vi "GateSTS v2.vi"(5 "Store\nSecond Gate?":bool=TRUE, 6 "Attributes":string[][](array[string]), 7 "Increment Gate (V)":dbl, 8 "End Gate (V)":dbl, 9 "Start Gate (V)":dbl, 10 "Basename":string) -> (3 "Stop Loop":bool)   [LabVIEW 2021]
uses:
  <userlib>/Nanonis Prog Interface V5/Nanonis Prog Interface.lvlib
panel:
  in  "Tabs":T1(tab)
  in  "Sweep second gate?":bool
  out "Sweep time (min)":dbl
  in  "Nanonis LI      Ext LI":bool=TRUE
  in  "Single spectrum?":bool
  in  "Time Constant (s)":T2(ring)=enum."10 ms"
  in  "Frequency (Hz)":dbl=1541.2 format="%#_6p"
  in  "End Bias (V)":dbl=0.04 format="%#_6p"
  in  "Start Bias (V)":dbl=-0.04 format="%#_6p"
  in  "Energy resolution (V)":dbl=0.001 format="%#_6p"
  in  "Stop":bool
  out "Current Gate Voltage (V)":dbl
  in  "?":bool
  out "HDF5 DATANAME":string
  in  "Run lockin?":bool=TRUE
  in  "Store\nLock-in\nParameters?":bool=TRUE
  in  "Store\nTemperatures?":bool
  in  "Store\nMagnetic Field?":bool
  in  "Zigzag Raster?":bool
  in  "Insert Loop Index\ninto Basename?":bool
  in  "Loop Forever?":bool
  out "Loop Index":i32
  in  "Loop Index Offset":i32=1
  in  "Make .dat files?":bool=TRUE
  out "Ender":bool
  # "Gate STS"
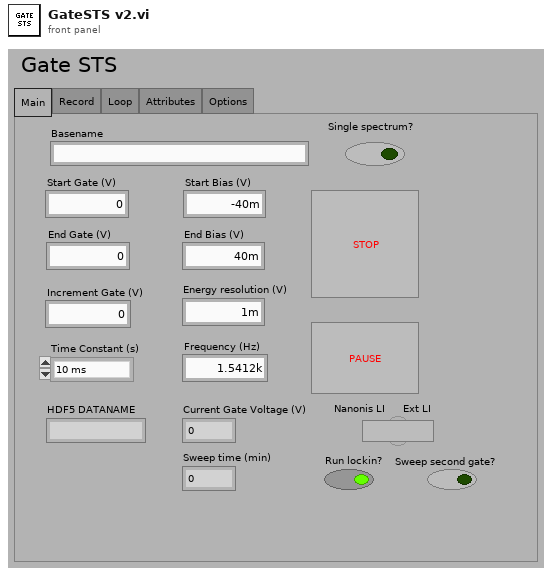
[diagram p1: front panel]
types:
  T1 = enum32{"Main", "Record", "Loop", "Attributes", "Options"}
  T2 = enum16{"10 us", "30 us", "100 us", "300 us", "1 ms", "3 ms", "10 ms", "30 ms", "100 ms", "300 ms", "1 s", "3 s", "10 s", "30 s", "100 s", "300 s", "1 ks", "3 ks", "10 ks", "30 ks"}
  T3 = enum16{"Set Amplitude", "Get Amplitude", "Set Frequency", "Get Frequency", "Set Harmonic", "Get Harmonic", "Set Phase", "Get Phase", "Auto Phase", "Add to Phase", "Autogain", "Set Time Constant", "Get Time Constant", "Set Sensitivity", "Get Sensitivity", "Set Input A", "Set Input A-B", "Get Input Setting", "Set Offset", "Get Offset"}
  T4 = cluster{"Save all":enum16{"no change", "on", "off"}, "Number of Sweeps (0=no change)":i32}
  T5 = enum16{"Set Voltage", "Read Voltage", "Read Current", "Output On", "Output Off", "Set Increment", "Set Increment Time", "Stop Voltage Set", "Set Maximum Voltage", "Get Maximum Voltage"}
  T6 = enum16{"Output 2 (V)", "Output 3 (V)", "Output 4 (V)"}
  T7 = enum16{"Read State", "Hold", "Ramp to Set", "Ramp to Zero", "Read Switch Heater", "Switch Heater On", "Switch Heater Off", "Read Voltage", "Read Current", "Read Field", "Read Persistent Field", "Read Target Field", "Set Target Field", "Read Ramp Rate", "Set Ramp Rate"}
  T8 = enum16{"pot_temp", "sorb_temp", "needle_valve_temp", "still_temp", "mix_chamber_temp", "stm_rx_temp", "stm_cx_temp", "tank_pressure", "condense_pressure", "still_pressure", "turbo_back_pressure", "n2_trap_pressure"}
  T9 = enum16{"Set Amplitude", "Get Amplitude", "Set Frequency", "Get Frequency", "Set Harmonic", "Get Harmonic", "Set Phase", "Get Phase", "Auto Phase", "Add to Phase", "Autogain", "Set Time Constant", "Get Time Constant", "Set Sensitivity", "Get Sensitivity", "Set Input A", "Set Input A-B", "Get Input Setting", "Set Offset", "Get Offset"}[]
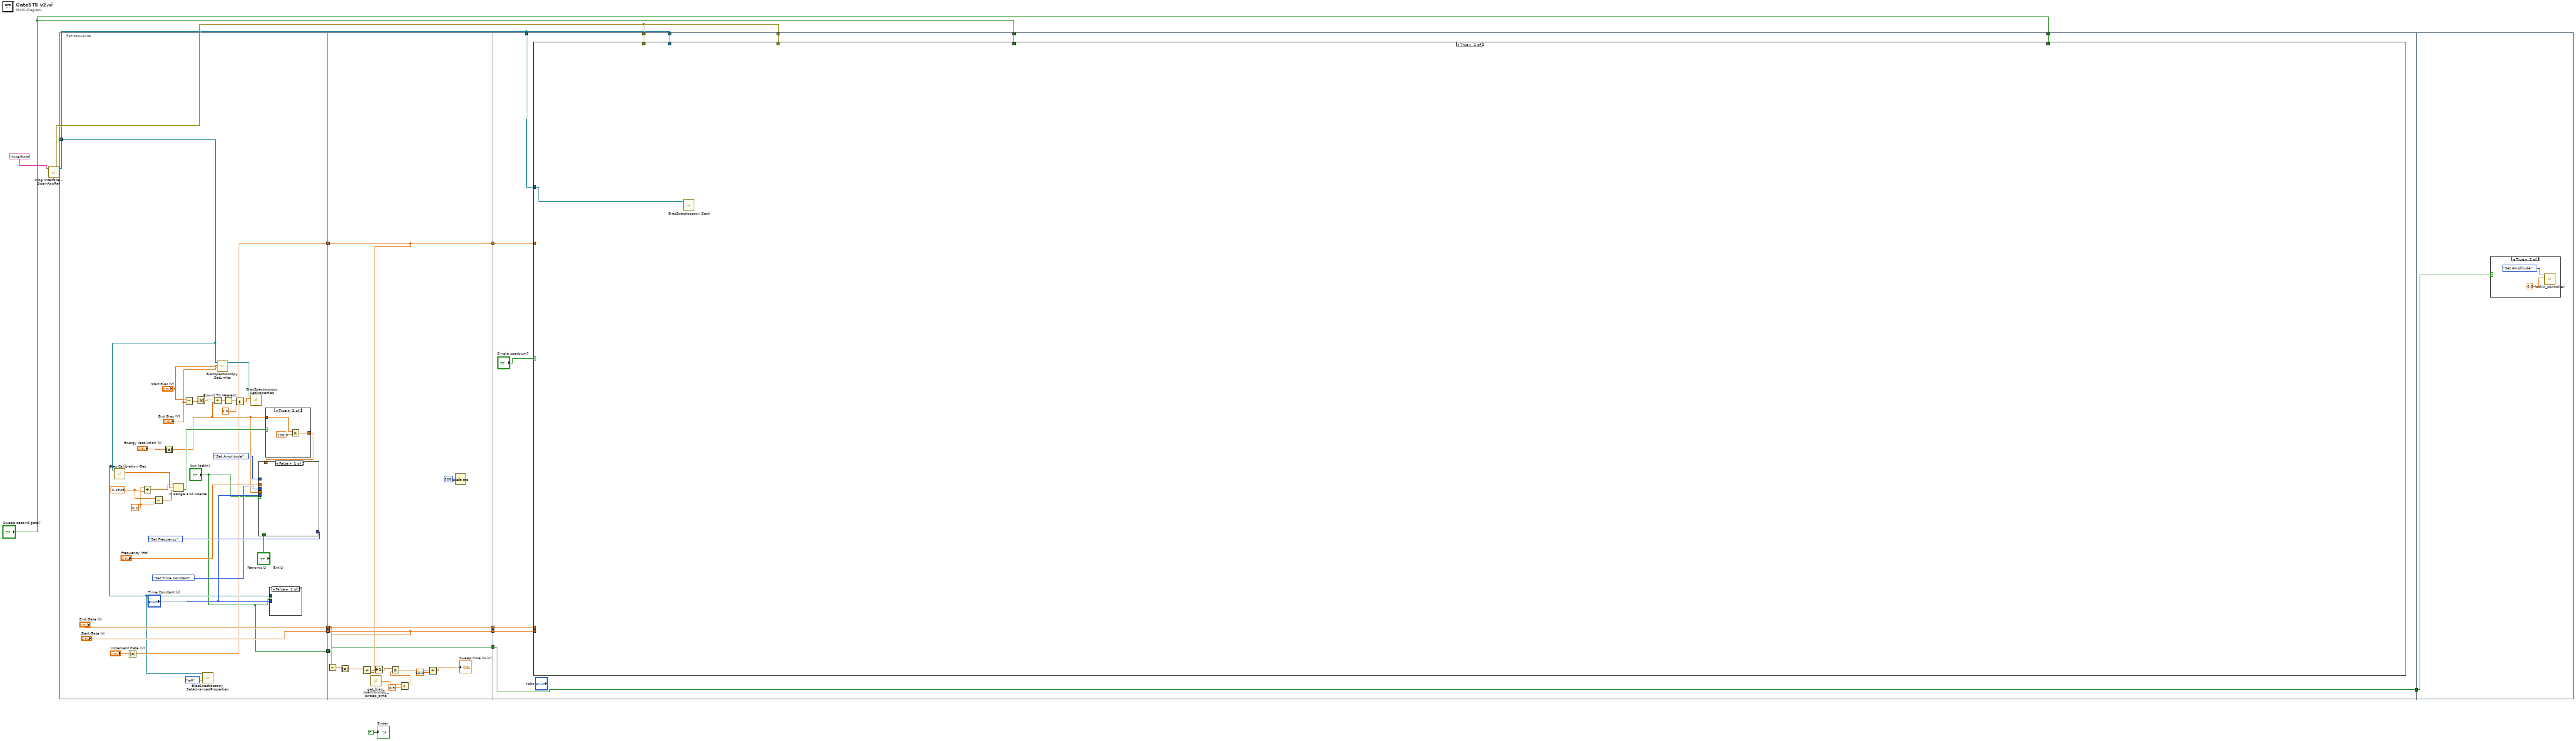
[diagram p0: block diagram]
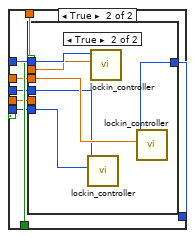
[diagram p2: hidden frame]
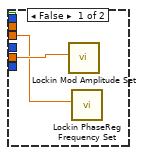
[diagram p3: hidden frame]
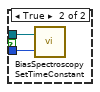
[diagram p4: hidden frame]
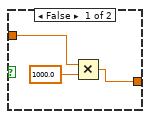
[diagram p5: hidden frame]
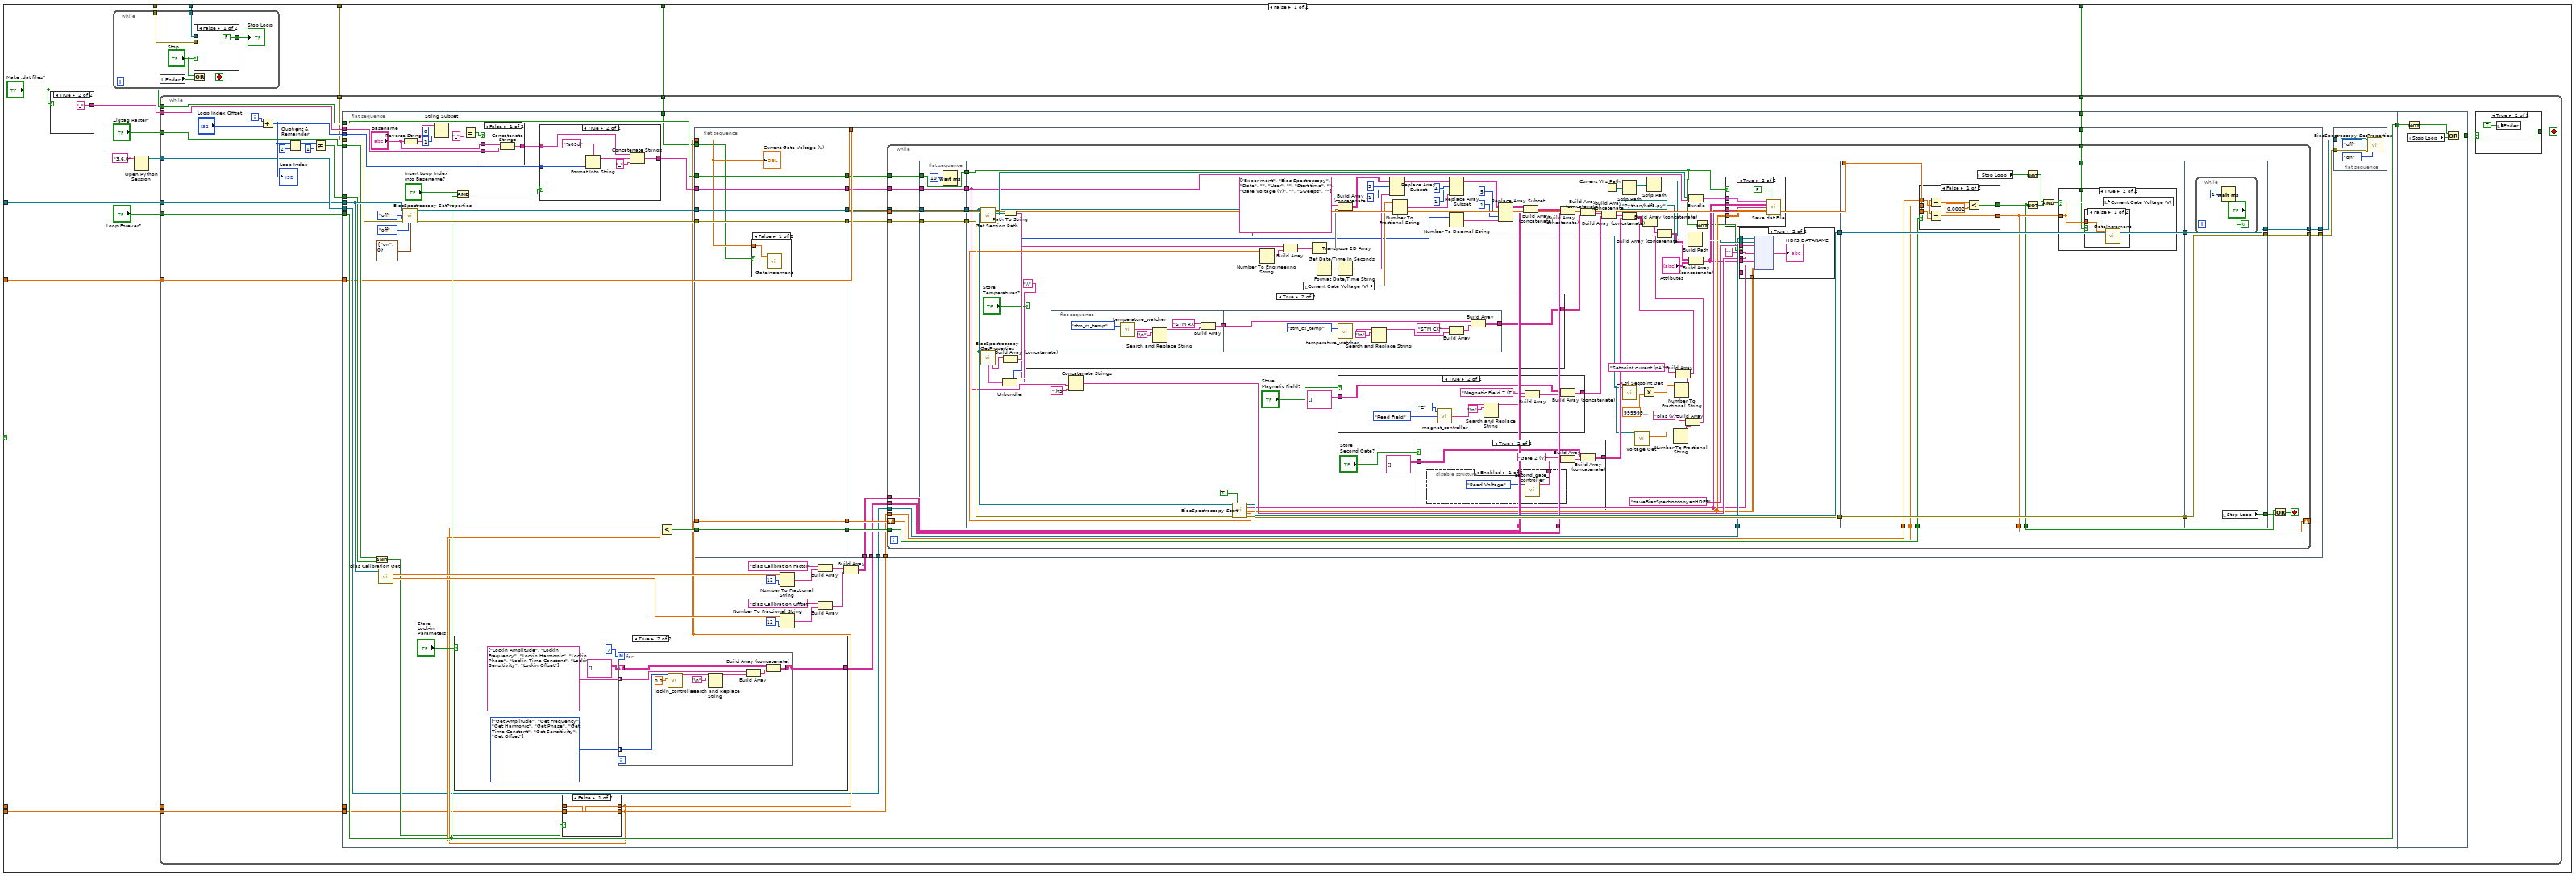
[diagram p6: hidden frame]
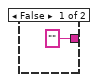
[diagram p7: hidden frame]
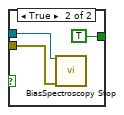
[diagram p8: hidden frame]
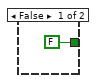
[diagram p9: hidden frame]
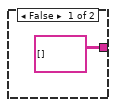
[diagram p13: hidden frame]
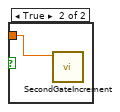
[diagram p14: hidden frame]
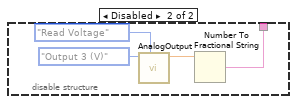
[diagram p17: hidden frame]
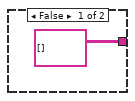
[diagram p20: hidden frame]
diagram:
  n1 = call <userlib>:"Prog Interface - OpenAppRef.vi"("Machine name (local machine IP)"="localhost" ("machine name (localhost)")) -> ("Error out"=w12:errorcluster, "Application reference"=w11:refnum<vi>)  [unwired: 5 in]
  n2 = flat-sequence {
    tunnel: w11 -> [w17]
    tunnel: ["End Gate (V)"] -> w9
    tunnel: ["Start Gate (V)"] -> w7
    tunnel: [w20] -> w5
    tunnel: ["Run lockin?"] -> w3
    tunnel: [w73] -> w10
    tunnel: w9 -> [w73]
    tunnel: [w72] -> w8
    tunnel: w7 -> [w72]
    tunnel: [w74] -> w6
    tunnel: w5 -> [w74]
    tunnel: w3 -> [w70]
    tunnel: [w70] -> w2
    tunnel: w12 -> [w95]
    tunnel: w12 -> [w94]
    tunnel: w11 -> [w93]
    tunnel: w11 -> [w92]
    tunnel: w10 -> [w90]
    tunnel: w8 -> [w89]
    tunnel: w6 -> [w88]
    tunnel: "Sweep second gate?" -> [w87]
    tunnel: "Sweep second gate?" -> [w86]
    tunnel: w2 -> [w85]
    tunnel: [w85] -> w1
    tunnel: w1 -> [w465]
    frame #0 {
      w38 = 0.1 ("y")
      w39 = 0.4945 ("x")
      n3 = call <userlib>:"Bias Calibration Get.vi"("Application ref in"=w17) -> ("Calibration (V/V)"=w41:sgl)  [unwired: 7 in, 3 out]
      n4 = Absolute Value(x="Increment Gate (V)") -> (abs(x)=w20:dbl)
      n5 = Add(x=w39, y=w38) -> (x+y=w40:dbl)
      n6 = Subtract(x=w39, y=w38) -> (x-y=w37:dbl)
      n7 = Absolute Value(x="Energy resolution (V)") -> (abs(x)=w22:dbl)
      n8 = In Range and Coerce(upper limit=w40, x=w41, lower limit=w37) -> (In Range?=w36:bool)  [unwired: 1 out]
      n9 = Subtract(x="Start Bias (V)", y="End Bias (V)") -> (x-y=w45:dbl)
      n10 = Absolute Value(x=w45) -> (abs(x)=w44:dbl)
      n11 = call <userlib>:"BiasSpectroscopy SetAdvancedProperties.vi"("Application ref in"=w17, "Lockin run (no change)"=enum16{"no change", "on", "off"}."off") -> ()  [unwired: 12 in, 2 out]
      n12 = Divide(x=w44, y=w22) -> (x/y=w43:dbl)
      n13 = call <userlib>:"BiasSpectroscopy SetLimits.vi"("End value (V)"="End Bias (V)", "Start value (V)"="Start Bias (V)", "Application ref in"=w17) -> ("Application ref out"=w42:refnum<vi>)  [unwired: 5 in, 1 out]
      n14 = Round To Nearest(number=w43) -> (nearest integer value=w33:dbl)
      n15 = Add(x=w33, y=1.0) -> (x+y=w31:dbl)
      n16 = call <userlib>:"BiasSpectroscopy SetProperties.vi"("Application ref in"=w42, "Number of points (0=no change)"=w31) -> ()  [unwired: 12 in, 2 out]
      n17 = case shown="True" w36 {
        tunnel: w22 -> [w65 w68]
        tunnel: [w64 w67] -> w34
        frame False {
          n18 = Multiply(x=w65, y=1000.0) -> (x*y=w64:dbl)
        }
        frame True {
          n19 = Multiply(x=w68, y=100.0) -> (x*y=w67:dbl)
        }
      }
      n20 = case shown="False" "Run lockin?" {
        tunnel: T3."Set Amplitude" ("Command") -> [_ w53]
        tunnel: w34 -> [_ w52]
        tunnel: "Nanonis LI      Ext LI" -> [_ w51]
        tunnel: "Frequency (Hz)" -> [_ w50]
        tunnel: T3."Set Frequency" ("Command") -> [_ w49]
        tunnel: "Time Constant (s)" -> [_ w48]
        tunnel: T3."Set Time Constant" ("Command") -> [_ w47]
        tunnel: w22 -> [_ w46]
        frame False {
        }
        frame True {
          n21 = case shown="True" w51 {
            tunnel: w53 -> [_ w61]
            tunnel: w52 -> [_ w60]
            tunnel: w50 -> [w54 w59]
            tunnel: w49 -> [_ w58]
            tunnel: w48 -> [_ w57]
            tunnel: w47 -> [_ w56]
            tunnel: w46 -> [w55 _]
            frame False {
              n22 = call <userlib>:"Lockin Mod Amplitude Set.vi"("Amplitude (mod. signal unit)"=w55) -> ()  [unwired: 9 in, 2 out]
              n23 = call <userlib>:"Lockin PhaseReg Frequency Set.vi"("Frequency (Hz)"=w54) -> ()  [unwired: 9 in, 2 out]
            }
            frame True {
              n24 = call "lockin_controller.vi"("Numerical Argument"=w57, "Command"=w56) -> ()  [unwired: 9 in, 1 out]
              n25 = call "lockin_controller.vi"("Numerical Argument"=w60, "Command"=w61) -> ()  [unwired: 9 in, 1 out]
              n26 = call "lockin_controller.vi"("Numerical Argument"=w59, "Command"=w58) -> ()  [unwired: 9 in, 1 out]
            }
          }
        }
      }
      n27 = case shown="False" "Run lockin?" {
        tunnel: w17 -> [_ w63]
        tunnel: "Time Constant (s)" -> [_ w62]
        frame False {
        }
        frame True {
          n28 = call "BiasSpectroscopySetTimeConstant.vi"("Set Time Constant"=w62, "Application ref in"=w63) -> ()  [unwired: 1 in, 1 out]
        }
      }
    }
    frame #1 {
      n29 = Subtract(x=w72, y=w73) -> (x-y=w77:dbl)
      n30 = Absolute Value(x=w77) -> (abs(x)=w78:dbl)
      n31 = Divide(x=w78, y=w74) -> (x/y=w79:dbl)
      n32 = call "get_bias_spectroscopy_sweep_time.vi"() -> ("Sweep time (s)"=w81:sgl)
      n33 = Increment(x=w79) -> (x+1=w80:dbl)
      n34 = Add(x=w81, y=sgl 0.5) -> (x+y=w82:sgl)
      n35 = Multiply(x=w80, y=w82) -> (x*y=w83:dbl)
      n36 = Divide(x=w83, y=60.0) -> (x/y=→"Sweep time (min)":dbl)
      n37 = Wait (ms)(milliseconds to wait=u32 500) -> ()  [unwired: 1 out]
    }
    frame #2 {
      n38 = case shown="True" "Single spectrum?" {
        tunnel: w95 -> [w104 _]
        tunnel: w94 -> [w103 _]
        tunnel: w93 -> [w102 _]
        tunnel: w92 -> [w101 w464]
        tunnel: w90 -> [w100 _]
        tunnel: w89 -> [w99 _]
        tunnel: w88 -> [w98 _]
        tunnel: w87 -> [w97 _]
        tunnel: w86 -> [w96 _]
        frame False {
          n39 = case shown="True" "Make .dat files?" {
            tunnel: ["" ("string") "_" ("string")] -> w106
            frame False {
            }
            frame True {
            }
          }
          n40 = while {
            tunnel: w104 -> [w114]
            tunnel: w102 -> [w113]
            stop <- w116 stop-if-true
            n41 = local read "Ender"() -> (w115:bool)
            n42 = Or(x="Stop", y=w115) -> (x .or. y?=w116:bool)
            n43 = case shown="False" "Stop" {
              tunnel: w113 -> [_ w122]
              tunnel: w114 -> [_ w121]
              tunnel: [FALSE TRUE] -> w118
              frame False {
              }
              frame True {
                n44 = call <userlib>:"BiasSpectroscopy Stop.vi"("Application ref in"=w122, "Error in (no error)"=w121) -> ()  [unwired: 12 in, 2 out]
              }
            }
            "Stop Loop" <- w118
          }
          n45 = Open Python Session(python version="3.6.0" ("Python version")) -> (session out=w108:refnum<k35>)  [unwired: 2 in, 1 out]
          n46 = while {
            tunnel: "Loop Forever?" -> [w144]
            tunnel: "Zigzag Raster?" -> [w139]
            tunnel: w108 -> [w132]
            tunnel: w106 -> [w131]
            tunnel: "Make .dat files?" -> [w130]
            tunnel: w103 -> [w129]
            tunnel: w101 -> [w128]
            tunnel: w100 -> [w127]
            tunnel: w99 -> [w126]
            tunnel: w98 -> [w125]
            tunnel: w97 -> [w124]
            tunnel: w96 -> [w123]
            i -> [w140]
            stop <- w141 stop-if-true
            n47 = Add(x=w140, y="Loop Index Offset") -> (x+y=w137:i32)
            "Loop Index" <- w137
            n48 = Quotient & Remainder(x=w137, y=2) -> (x-y*floor(x/y)=w135:i32)  [unwired: 1 out]
            n49 = Not Equal?(x=w135, y=1) -> (x != y?=w133:bool)
            n50 = flat-sequence {
              tunnel: w144 -> [w172]
              tunnel: [w172] -> w143
              tunnel: w128 -> [w176]
              tunnel: w129 -> [w175]
              tunnel: w137 -> [w170]
              tunnel: w139 -> [w159]
              tunnel: w133 -> [w158]
              tunnel: w132 -> [w156]
              tunnel: w131 -> [w155]
              tunnel: w130 -> [w153]
              tunnel: w127 -> [w152]
              tunnel: w126 -> [w151]
              tunnel: w125 -> [w150]
              tunnel: w124 -> [w149]
              tunnel: w123 -> [w148]
              tunnel: w143 -> [w463]
              tunnel: [w460] -> w142
              frame #0 {
                n51 = And(x=w159, y=w158) -> (x .and. y?=w157:bool)
                n52 = call <userlib>:"Bias Calibration Get.vi"("Application ref in"=w176) -> ("Offset (V)"=w186:sgl, "Calibration (V/V)"=w187:sgl)  [unwired: 7 in, 2 out]
                n53 = Reverse String(1:"Basename") -> (0:w167:string)
                n54 = call <userlib>:"BiasSpectroscopy SetProperties.vi"("Application ref in"=w176, "Autosave (no change)"=enum16{"no change", "on", "off"}."off", "Error in (no error)"=w175, "Save dialog"=enum16{"no change", "on", "off"}."off", "Multiple sweeps config"=T4 {"Save all"=enum."on", "Number of Sweeps (0=no change)"=0}) -> ("Application ref out"=w196:refnum<vi>, "Error out"=w197:errorcluster)  [unwired: 9 in]
                n55 = String Subset(string=w167, offset (0)=0, length (rest)=1 ("length (rest)")) -> (substring=w166:string)
                n56 = case shown="True" "Store\nLock-in\nParameters?" {
                  tunnel: [string[][] [] w219] -> w188
                  frame False {
                  }
                  frame True {
                    w222 = T9 [enum."Get Amplitude", enum."Get Frequency", enum."Get Harmonic", enum."Get Phase", enum."Get Time Constant", enum."Get Sensitivity", enum."Get Offset"] items=["Set Amplitude", "Get Amplitude", "Set Frequency", "Get Frequency", "Set Harmonic", "Get Harmonic", "Set Phase", "Get Phase", "Auto Phase", "Add to Phase", "Autogain", "Set Time Constant", "Get Time Constant", "Set Sensitivity", "Get Sensitivity", "Set Input A", "Set Input A-B", "Get Input Setting", "Set Offset", "Get Offset"]
                    n57 = for {
                      N: 7 -> [_]
                      tunnel: w222 -> [w230] mode=indexing
                      tunnel: string[] ["Lockin Amplitude", "Lockin Frequency", "Lockin Harmonic", "Lockin Phase", "Lockin Time Constant", "Lockin Sensitivity", "Lockin Offset"] -> [w229] mode=indexing
                      shift-right: [w227] -> w219
                      shift-left: string[][] [] -> [w228]
                      n58 = call "lockin_controller.vi"("Numerical Argument"=0.0, "Command"=w230) -> ("Response"=w225:string)  [unwired: 9 in]
                      n59 = Search and Replace String(input string=w225, search string="\n") -> (result string=w226:string)  [unwired: 6 in, 3 out]
                      n60 = Build Array(w229, w226) -> (w231:string[])
                      n61 = Build Array (concatenate)(w228, w231) -> (w227:string[][])
                    }
                  }
                }
                n62 = And(x="Insert Loop Index\ninto Basename?", y=w172) -> (x .and. y?=w171:bool)
                n63 = Equal?(x=w166, y="_") -> (x = y?=w164:bool)
                n64 = case shown="False" w164 {
                  tunnel: "Basename" -> [w209 w210]
                  tunnel: [w208 w210] -> w162
                  tunnel: w155 -> [w207 _]
                  frame False {
                    n65 = Concatenate Strings(w209, w207) -> (w208:string)
                  }
                  frame True {
                  }
                }
                n66 = case shown="True" w171 {
                  tunnel: [w211 w217] -> w174
                  tunnel: w162 -> [w211 w216]
                  tunnel: w170 -> [_ w214]
                  frame False {
                  }
                  frame True {
                    n67 = Format Into String(format string="%05d", w214) -> (resulting string=w212:string)  [unwired: 2 in, 1 out]
                    n68 = Concatenate Strings(w216, w212, "_" ("string")) -> (w217:string)
                  }
                }
                n69 = case shown="False" w157 {
                  tunnel: w152 -> [w204 w206]
                  tunnel: [w204 w205] -> w161
                  tunnel: [w203 w206] -> w160
                  tunnel: w151 -> [w203 w205]
                  frame False {
                  }
                  frame True {
                  }
                }
                n70 = Less?(x=w160, y=w161) -> (x < y?=w191:bool)
                n71 = flat-sequence {
                  tunnel: w160 -> [w240]
                  tunnel: w191 -> [w241]
                  tunnel: w196 -> [w242]
                  tunnel: w197 -> [w243]
                  tunnel: w174 -> [w244]
                  tunnel: [w244] -> w202
                  tunnel: [w243] -> w201
                  tunnel: [w242] -> w200
                  tunnel: [w241] -> w199
                  tunnel: [w240] -> w198
                  tunnel: w160 -> [w239]
                  tunnel: [w238] -> w154
                  tunnel: w153 -> [w238]
                  tunnel: w149 -> [w237]
                  tunnel: [w257] -> w194
                  tunnel: [w256] -> w193
                  tunnel: w202 -> [w260]
                  tunnel: w201 -> [w259]
                  tunnel: w200 -> [w258]
                  tunnel: w199 -> [w255]
                  tunnel: w198 -> [w254]
                  tunnel: w161 -> [w253]
                  tunnel: w188 -> [w252]
                  tunnel: w177 -> [w251]
                  tunnel: w156 -> [w250]
                  tunnel: w154 -> [w249]
                  tunnel: w150 -> [w248]
                  tunnel: w148 -> [w247]
                  frame #0 {
                    n72 = case shown="False" w237 {
                      tunnel: w239 -> [w245 w246]
                      frame False {
                        n73 = call "GateIncrement.vi"("Gate Voltage"=w245) -> ()  [unwired: 11 in]
                      }
                      frame True {
                        n74 = call "SecondGateIncrement.vi"("Gate Voltage"=w246) -> ()  [unwired: 11 in]
                      }
                    }
                    "Current Gate Voltage (V)" <- w239
                  }
                  frame #1 {
                    n75 = while {
                      tunnel: w260 -> [w286]
                      tunnel: w259 -> [w285]
                      tunnel: w258 -> [w284]
                      tunnel: [w283] -> w257
                      tunnel: [w282] -> w256
                      tunnel: w255 -> [w268]
                      shift-right: [w272] -> _
                      shift-left: w254 -> [w270]
                      tunnel: w253 -> [w269]
                      tunnel: w252 -> [w267]
                      tunnel: w251 -> [w266]
                      tunnel: w250 -> [w265]
                      tunnel: w249 -> [w263]
                      tunnel: w248 -> [w262]
                      tunnel: w247 -> [w261]
                      stop <- w273 stop-if-true
                      n76 = flat-sequence {
                        tunnel: w284 -> [w289]
                        tunnel: w285 -> [w290]
                        tunnel: w286 -> [w291]
                        tunnel: [w291] -> w277
                        tunnel: [w290] -> w276
                        tunnel: [w289] -> w275
                        tunnel: [w287] -> w264
                        tunnel: w263 -> [w287]
                        tunnel: [w368] -> w279
                        tunnel: [w369] -> w278
                        tunnel: w277 -> [w325]
                        tunnel: w276 -> [w370]
                        tunnel: w275 -> [w366]
                        tunnel: w267 -> [w341]
                        tunnel: w266 -> [w339]
                        tunnel: w265 -> [w328]
                        tunnel: w264 -> [w292]
                        tunnel: [w436] -> w281
                        tunnel: [w435] -> w280
                        tunnel: w279 -> [w436]
                        tunnel: w278 -> [w435]
                        tunnel: [w431] -> w272
                        tunnel: [w429] -> w271
                        tunnel: w270 -> [w428]
                        tunnel: w269 -> [w427]
                        tunnel: w268 -> [w426]
                        tunnel: w262 -> [w425]
                        tunnel: w261 -> [w424]
                        tunnel: [w456] -> w283
                        tunnel: [w457] -> w282
                        tunnel: w281 -> [w457]
                        tunnel: w280 -> [w456]
                        tunnel: [w455] -> w274
                        frame #0 {
                          n77 = Wait (ms)(milliseconds to wait=u32 10) -> ()  [unwired: 1 out]
                        }
                        frame #1 {
                          n78 = call <userlib>:"Get Session Path.vi"("Application ref in"=w366) -> ("Session path"=w326:path, "Application ref out"=w300:refnum<vi>)  [unwired: 8 in, 1 out]
                          n79 = call <userlib>:"BiasSpectroscopy GetProperties.vi"("Application ref in"=w366) -> ("Parameters"=w358:string[], "Multiple sweeps configuration"=w347:cluster{"Number of Sweeps":i32, "Save all":bool}, "Fixed parameters"=w359:string[])  [unwired: 7 in, 5 out]
                          n80 = Unbundle(w347) -> ("Number of Sweeps"=w346:i32)  [unwired: 1 out]
                          n81 = Path To String(path=w326) -> (string=w319:string)
                          n82 = Build Array (concatenate)(w359, w358) -> (w363:string[])
                          n83 = case shown="True" "Store\nTemperatures?" {
                            tunnel: [string[][] [] w408] -> w335
                            frame False {
                            }
                            frame True {
                              n84 = flat-sequence {
                                tunnel: [w413] -> w409
                                tunnel: w409 -> [w420]
                                tunnel: [w419] -> w408
                                frame #0 {
                                n85 = call "temperature_watcher.vi"("Command"=T8."stm_rx_temp") -> ("Response"=w411:string)  [unwired: 1 in]
                                n86 = Search and Replace String(input string=w411, search string="\n") -> (result string=w410:string)  [unwired: 6 in, 3 out]
                                n87 = Build Array("STM RX" ("element"), w410) -> (w413:string[])
                                }
                                frame #1 {
                                n88 = call "temperature_watcher.vi"("Command"=T8."stm_cx_temp") -> ("Response"=w417:string)  [unwired: 1 in]
                                n89 = Search and Replace String(input string=w417, search string="\n") -> (result string=w416:string)  [unwired: 6 in, 3 out]
                                n90 = Build Array("STM CX" ("element"), w416) -> (w421:string[])
                                n91 = Build Array(w420, w421) -> (w419:string[][])
                                }
                              }
                            }
                          }
                          n92 = Concatenate Strings(w319, "\\" ("string"), w325, ".h5" ("string")) -> (w323:string)
                          n93 = call <userlib>:"BiasSpectroscopy Start.vi"("Application ref in"=w366, "Get data (F)"=TRUE, "Error in (no error)"=w370) -> ("Application ref out"=w369:refnum<vi>, "Channels"=w316:string[], "Data"=w317:sgl[][], "Parameters"=w365:sgl[], "Error out"=w368:errorcluster)  [unwired: 8 in]
                          n94 = Number To Engineering String(4:w365) -> (0:w364:string[])  [unwired: 3 in]
                          n95 = Build Array(w363, w364) -> (w362:string[][])
                          n96 = local read "Current Gate Voltage (V)"() -> (w349:dbl)
                          n97 = Transpose 2D Array(2D array=w362) -> (transposed array=w360:string[][])
                          n98 = Get Date/Time In Seconds() -> (seconds since 1Jan1904=w357:timestamp)
                          n99 = Build Array (concatenate)(string[][] [["Experiment", "Bias Spectroscopy"], ["Date", ""], ["User", ""], ["Start time", ""], ["Gate Voltage (V)", ""], ["Sweeps", ""]] ("Attributes"), w360) -> (w356:string[][])
                          n100 = Format Date/Time String(seconds (now)=w357) -> (date/time string=w355:string)  [unwired: 2 in]
                          n101 = case shown="True" "Store\nMagnetic Field?" {
                            tunnel: [w397 w401] -> w332
                            tunnel: string[][] [] ("array") -> [w397 w402]
                            frame False {
                            }
                            frame True {
                              n102 = call "magnet_controller.vi"("Command"=T7."Read Field", "Direction"=enum16{"X", "Y", "Z"}."Z") -> ("Response"=w399:string)  [unwired: 1 in]
                              n103 = Search and Replace String(input string=w399, search string="\n") -> (result string=w398:string)  [unwired: 6 in, 3 out]
                              n104 = Build Array("Magnetic Field Z (T)" ("element"), w398) -> (w403:string[])
                              n105 = Build Array (concatenate)(w402, w403) -> (w401:string[][])
                            }
                          }
                          n106 = Replace Array Subset(array=w356, new element=w355, index (row)=3, index (col)=1 ("disabled index (col)")) -> (w352:string[][])
                          n107 = Number To Fractional String(number=w349) -> (F-format string=w348:string)  [unwired: 3 in]
                          n108 = case shown="True" "Store\nSecond Gate?" {
                            tunnel: [w380 w382] -> w308
                            tunnel: string[][] [] ("array") -> [w380 w383]
                            frame False {
                            }
                            frame True {
                              n109 = disable-structure shown="Enabled" {
                                disable-tunnel: [w387 w391] -> w381
                                frame Enabled {
                                n110 = call "second_gate_controller.vi"("Command"=T5."Read Voltage") -> ("Response"=w387:string)  [unwired: 10 in]
                                }
                                frame Disabled {
                                n111 = call "AnalogOutput.vi"("Read or Set Voltage?"=enum16{"Read Voltage", "Set Voltage"}."Read Voltage", "Channel"=T6."Output 3 (V)") -> ("Output Voltage"=w390:sgl)  [unwired: 9 in]
                                n112 = Number To Fractional String(number=w390) -> (F-format string=w391:string)  [unwired: 3 in]
                                }
                              }
                              n113 = Build Array("Gate 2 (V)" ("element"), w381) -> (w384:string[])
                              n114 = Build Array (concatenate)(w383, w384) -> (w382:string[][])
                            }
                          }
                          n115 = Replace Array Subset(array=w352, new element=w348, index (row)=4, index (col)=1 ("disabled index (col)")) -> (w345:string[][])
                          n116 = Number To Decimal String(number=w346) -> (decimal integer string=w342:string)  [unwired: 1 in]
                          n117 = Replace Array Subset(array=w345, new element=w342, index (row)=5, index (col)=1 ("disabled index (col)")) -> (w340:string[][])
                          n118 = Build Array (concatenate)(w340, w339) -> (w338:string[][])
                          n119 = Build Array (concatenate)(w338, w341) -> (w336:string[][])
                          n120 = Build Array (concatenate)(w336, w335) -> (w333:string[][])
                          n121 = Build Array (concatenate)(w333, w332) -> (w311:string[][])
                          n122 = Current VI's Path() -> (path=w320:path)
                          n123 = Strip Path(path=w320) -> (stripped path=w321:path)  [unwired: 1 out]
                          n124 = Build Array (concatenate)(w311, w308) -> (w307:string[][])
                          n125 = call <userlib>:"Z-Ctrl Setpoint Get.vi"("Application ref in"=w300) -> ("Z Controller setpoint"=w296:sgl)  [unwired: 7 in, 2 out]
                          n126 = call <userlib>:"Voltage Get.vi"("Application ref in"=w300) -> ("Bias (V)"=w301:sgl)  [unwired: 8 in, 2 out]
                          n127 = Multiply(x=w296, y=sgl 1000000000000.0) -> (x*y=w294:sgl)
                          n128 = Strip Path(path=w321) -> (stripped path=w322:path)  [unwired: 1 out]
                          n129 = Number To Fractional String(number=w301) -> (F-format string=w303:string)  [unwired: 3 in]
                          n130 = Number To Fractional String(number=w294) -> (F-format string=w306:string)  [unwired: 3 in]
                          n131 = Build Array("Setpoint current (pA)" ("element"), w306) -> (w304:string[])
                          n132 = Build Array (concatenate)(w307, w304) -> (w299:string[][])
                          n133 = Build Array("Bias (V)" ("element"), w303) -> (w298:string[])
                          n134 = Build Array (concatenate)(w299, w298) -> (w297:string[][])
                          n135 = Build Path(base path=w322, name or relative path=path "Python/hdf5.py") -> (appended path=w329:path)
                          n136 = Bundle("Session path"=w326, "Basename"=w325) -> (w315:cluster{"Session path":path, "Basename":string})  [unwired: 1 in]
                          n137 = Build Array (concatenate)(w297, "Attributes") -> (w312:string[][])
                          n138 = Not(x=w292) -> (.not. x?=w293:bool)
                          n139 = case shown="True" w292 {
                            tunnel: w312 -> [_ w396]
                            tunnel: w317 -> [_ w395]
                            tunnel: w316 -> [_ w394]
                            tunnel: w315 -> [_ w393]
                            frame False {
                            }
                            frame True {
                              n140 = call <userlib>:"Save dat File.vi"("Filename control"=w393, "Show save dialog (T)"=FALSE, "Attributes"=w396, "Channels names"=w394, "Data"=w395) -> ()  [unwired: 7 in, 4 out]
                            }
                          }
                          n141 = case shown="True" w293 {
                            tunnel: w329 -> [_ w379]
                            tunnel: w328 -> [_ w378]
                            tunnel: "saveBiasSpectroscopyasHDF5" ("function name") -> [_ w377]
                            tunnel: w323 -> [_ w376]
                            tunnel: w317 -> [_ w375]
                            tunnel: w316 -> [_ w374]
                            tunnel: "" ("function name") -> [_ w373]
                            tunnel: w312 -> [_ w371]
                            frame False {
                            }
                            frame True {
                              n142 = node(w378, w379, w377, w373, w376, w371, w374, w375) -> (→"HDF5 DATANAME":string)  [unwired: 5 in, 4 out]
                            }
                          }
                        }
                        frame #2 {
                          n143 = case shown="False" w426 {
                            tunnel: w428 -> [w441 w447]
                            tunnel: w425 -> [w442 w450]
                            tunnel: [w443 w449] -> w431
                            tunnel: w427 -> [w440 w448]
                            tunnel: [w438 w446] -> w429
                            frame False {
                              n144 = Subtract(x=w441, y=w440) -> (x-y=w439:dbl)
                              n145 = Subtract(x=w441, y=w442) -> (x-y=w443:dbl)
                              n146 = Less?(x=w439, y=0.0002) -> (x < y?=w438:bool)
                            }
                            frame True {
                              n147 = Subtract(x=w447, y=w448) -> (x-y=w445:dbl)
                              n148 = Add(x=w447, y=w450) -> (x+y=w449:dbl)
                              n149 = Greater?(x=w445, y=-0.0002) -> (0:w446:bool)
                            }
                          }
                          n150 = local read "Stop Loop"() -> (w434:bool)
                          n151 = Not(x=w434) -> (.not. x?=w432:bool)
                          n152 = Not(x=w429) -> (.not. x?=w430:bool)
                          n153 = And(x=w432, y=w430) -> (x .and. y?=w433:bool)
                          n154 = case shown="True" w433 {
                            tunnel: w431 -> [_ w452]
                            tunnel: w424 -> [_ w451]
                            frame False {
                            }
                            frame True {
                              n155 = case shown="False" w451 {
                                tunnel: w452 -> [w453 w454]
                                frame False {
                                n156 = call "GateIncrement.vi"("Gate Voltage"=w453) -> ()  [unwired: 11 in]
                                }
                                frame True {
                                n157 = call "SecondGateIncrement.vi"("Gate Voltage"=w454) -> ()  [unwired: 11 in]
                                }
                              }
                              n158 = local write "Current Gate Voltage (V)"(w452) -> ()
                            }
                          }
                        }
                        frame #3 {
                          n159 = while {
                            stop <- "?" continue-if-true
                            n160 = Wait (ms)(milliseconds to wait=u32 1) -> ()  [unwired: 1 out]
                          }
                          n161 = local read "Stop Loop"() -> (w455:bool)
                        }
                      }
                      n162 = Or(x=w271, y=w274) -> (x .or. y?=w273:bool)
                    }
                  }
                }
                n163 = Number To Fractional String(number=w187, precision (6)=i16 12) -> (F-format string=w183:string)  [unwired: 2 in]
                n164 = Number To Fractional String(number=w186, precision (6)=i16 12) -> (F-format string=w180:string)  [unwired: 2 in]
                n165 = Build Array("Bias Calibration Factor" ("element"), w183) -> (w178:string[])
                n166 = Build Array("Bias Calibration Offset" ("element"), w180) -> (w179:string[])
                n167 = Build Array(w178, w179) -> (w177:string[][])
                n168 = flat-sequence {
                  tunnel: w194 -> [w236]
                  tunnel: w193 -> [w235]
                  frame #0 {
                    n169 = call <userlib>:"BiasSpectroscopy SetProperties.vi"("Application ref in"=w236, "Autosave (no change)"=enum16{"no change", "on", "off"}."off", "Error in (no error)"=w235, "Save dialog"=enum16{"no change", "on", "off"}."on") -> ()  [unwired: 10 in, 2 out]
                  }
                }
              }
              frame #1 {
                n170 = Not(x=w463) -> (.not. x?=w461:bool)
                n171 = local read "Stop Loop"() -> (w462:bool)
                n172 = Or(x=w461, y=w462) -> (x .or. y?=w460:bool)
              }
            }
            n173 = case shown="True" w142 {
              selector: w142 -> [_ w147]
              tunnel: [FALSE w147] -> w141
              frame False {
              }
              frame True {
                n174 = local write "Ender"(TRUE ("Ender")) -> ()
              }
            }
          }
        }
        frame True {
          n175 = call <userlib>:"BiasSpectroscopy Start.vi"("Application ref in"=w464) -> ()  [unwired: 10 in, 5 out]
        }
      }
    }
    frame #3 {
      n176 = case shown="True" w465 {
        frame False {
        }
        frame True {
          n177 = call "lockin_controller.vi"("Numerical Argument"=0.0, "Command"=T3."Set Amplitude") -> ()  [unwired: 9 in, 1 out]
        }
      }
    }
  }
  "Ender" <- FALSE ("Ender")
